vi "PM100D_SetRngIndex.vi"(5 "VISAin":refnum<visa-resource-name>, 7 "Unit":string, 9 "AUTO":bool, 11 "error in":errorcluster, 12 "SensType":i32, 13 "Rng_Array":string[](array[string]), 14 "Index":i32) -> (4 "VISAout":refnum<visa-resource-name>, 6 "lblRange":string, 8 "Numeric 2":dbl, 10 "AUTO?":bool, 15 "error out 2":errorcluster)   [LabVIEW 2015]
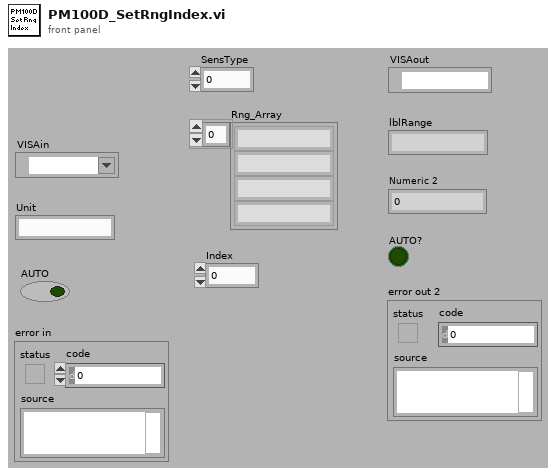
[diagram p1: front panel]
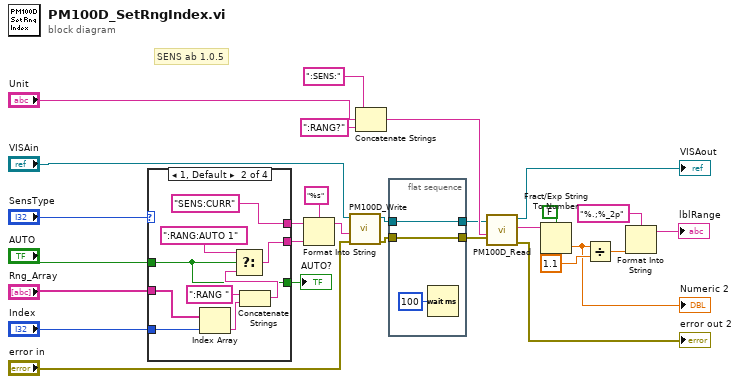
[diagram p0: block diagram]
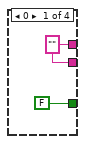
[diagram p2: hidden frame]
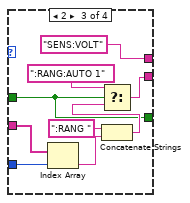
[diagram p3: hidden frame]
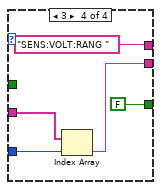
[diagram p4: hidden frame]
diagram:
  # "SENS ab 1.0.5"
  n1 = case shown="1, Default" "SensType" {
    tunnel: [w30 "SENS:CURR" "SENS:VOLT" "SENS:VOLT:RANG " ("string")] -> w15
    tunnel: "Index" -> [_ w39 w48 w53]
    tunnel: "AUTO" -> [_ w31 w40 _]
    tunnel: [w30 w37 w46 w52] -> w17
    tunnel: "Rng_Array" -> [_ w36 w45 w51]
    tunnel: [FALSE ("AUTO") w31 w40 FALSE ("AUTO")] -> w25
    frame 0 {
      w30 = ""
    }
    frame 1, Default {
      n2 = Index Array(array=w36, index=w39) -> (element=w35:string)
      n3 = Concatenate Strings(":RANG " ("string"), w35) -> (w33:string)
      n4 = Select(t=":RANG:AUTO 1", s=w31, f=w33) -> (s? t:f=w37:string)
    }
    frame 2 {
      n5 = Index Array(array=w45, index=w48) -> (element=w42:string)
      n6 = Concatenate Strings(":RANG " ("string"), w42) -> (w41:string)
      n7 = Select(t=":RANG:AUTO 1", s=w40, f=w41) -> (s? t:f=w46:string)
    }
    frame 3 {
      n8 = Index Array(array=w51, index=w53) -> (element=w52:string)
    }
  }
  "AUTO?" <- w25
  n9 = Format Into String(format string="%s", initial string=w15, w17) -> (resulting string=w14:string)  [unwired: 1 in, 1 out]
  n10 = call "PM100D_Write.vi"("error in (no error)"="error in", "Command"=w14, "VISA in"="VISAin") -> ("error out"=w2:errorcluster, "VISA out"=w4:refnum<visa-resource-name>)  [unwired: 7 in]
  n11 = Concatenate Strings(":SENS:" ("string"), "Unit", ":RANG?" ("string")) -> (w18:string)
  n12 = flat-sequence {
    tunnel: [w56] -> w3
    tunnel: w4 -> [w56]
    tunnel: w2 -> [w55]
    tunnel: [w55] -> w1
    frame #0 {
      n13 = Wait (ms)(milliseconds to wait=u32 100) -> ()  [unwired: 1 out]
    }
  }
  n14 = call "PM100D_Read.vi"("error in (no error)"=w1, "Command"=w18, "VISA in"=w3) -> ("error out"=→"error out 2":errorcluster, "ReadValue"=w8:string, "VISA out"=→"VISAout":refnum<visa-resource-name>)  [unwired: 6 in]
  n15 = Fract/Exp String To Number(use system decimal point (T)=FALSE, string=w8) -> (number=w10:dbl)  [unwired: 2 in, 1 out]
  "Numeric 2" <- w10
  n16 = Divide(x=w10, y=1.1) -> (x/y=w12:dbl)
  n17 = Format Into String(format string="%.;%_2p", w12) -> (resulting string=→"lblRange":string)  [unwired: 2 in, 1 out]
